vi "Custom Error Codes.vi"(8 "error in":errorcluster, 10 "PAR1":string, 11 "Enum":T1) -> (0 "error out":errorcluster)   [LabVIEW 2013, in "GOLPI library.lvlib"]
uses:
  GOLPI library.lvlib
  Custom Error Codes Enum Type Def.vi
  <vilib>/Utility/error.llb/Error Cluster From Error Code.vi
  <vilib>/ErrorRing/Error Ring.xnode
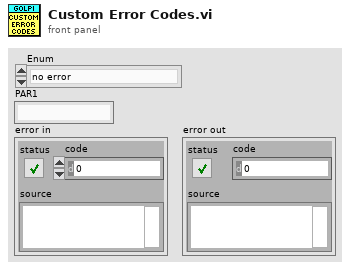
[diagram p1: front panel]
types:
  T1 = typedef "GOLPI library.lvlib/Custom Error Codes Enum Type Def.vi" = enum16{"no error", "00 working directory PAR1 missing", "01 octave binary PAR1 missing", "02 octave report error PAR1", "03 empty output last cmd PAR1", "10 var PAR1 not string", "11 var PAR1 not num, scal, ~compl", "12 var PAR1 not num, scal, compl", "13 var PAR1 not num, vect, ~compl", "14 var PAR1 not num, vect, compl"}
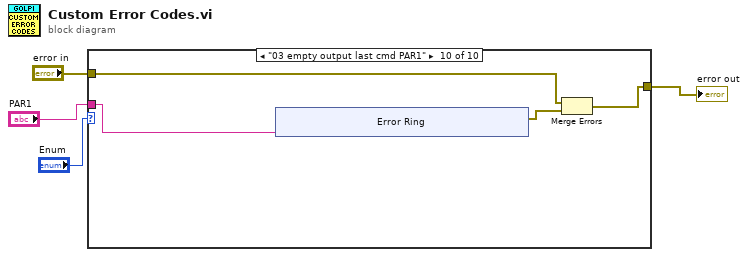
[diagram p0: block diagram]
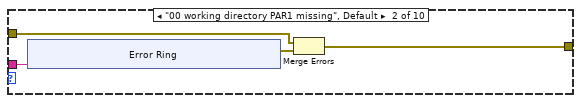
[diagram p3: hidden frame]
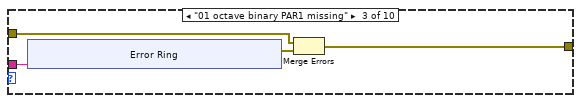
[diagram p4: hidden frame]
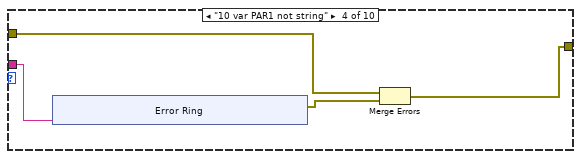
[diagram p5: hidden frame]
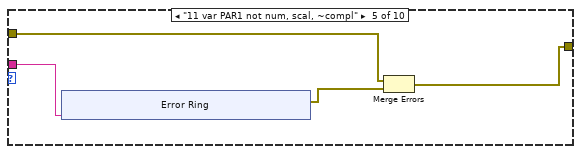
[diagram p6: hidden frame]
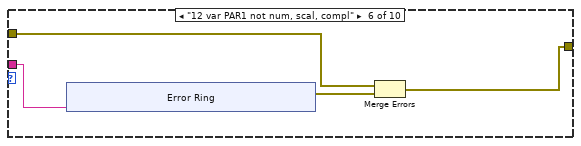
[diagram p7: hidden frame]
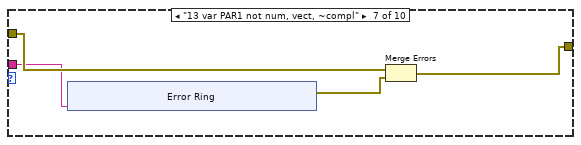
[diagram p8: hidden frame]
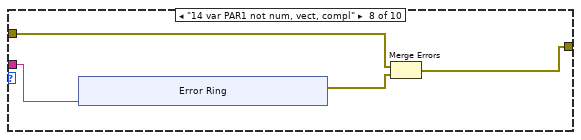
[diagram p9: hidden frame]
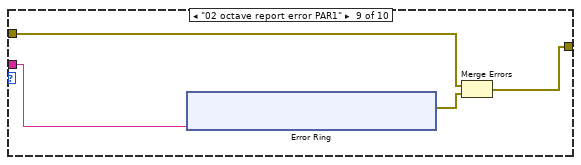
[diagram p10: hidden frame]
diagram:
  n1 = case shown="\"03 empty output last cmd PAR1\"" "Enum" {
    tunnel: "PAR1" -> [_ w9 w20 w28 w39 w51 w61 w73 w84 w97]
    tunnel: [w5 w7 w18 w29 w40 w50 w63 w72 w83 w94] -> w1
    tunnel: "error in" -> [w5 w6 w17 w30 w41 w53 w64 w74 w85 w95]
    frame "no error" {
    }
    frame "00 working directory PAR1 missing", Default {
      n2 = xnode "Error Ring"("parameter 0"=w9) -> ("error out"=w8:errorcluster)
      n3 = Merge Errors(w6, w8) -> (w7:errorcluster)
    }
    frame "01 octave binary PAR1 missing" {
      n4 = xnode "Error Ring"("parameter 0"=w20) -> ("error out"=w19:errorcluster)
      n5 = Merge Errors(w17, w19) -> (w18:errorcluster)
    }
    frame "10 var PAR1 not string" {
      n6 = xnode "Error Ring"("parameter 0"=w28) -> ("error out"=w31:errorcluster)
      n7 = Merge Errors(w30, w31) -> (w29:errorcluster)
    }
    frame "11 var PAR1 not num, scal, ~compl" {
      n8 = xnode "Error Ring"("parameter 0"=w39) -> ("error out"=w42:errorcluster)
      n9 = Merge Errors(w41, w42) -> (w40:errorcluster)
    }
    frame "12 var PAR1 not num, scal, compl" {
      n10 = xnode "Error Ring"("parameter 0"=w51) -> ("error out"=w52:errorcluster)
      n11 = Merge Errors(w53, w52) -> (w50:errorcluster)
    }
    frame "13 var PAR1 not num, vect, ~compl" {
      n12 = xnode "Error Ring"("parameter 0"=w61) -> ("error out"=w62:errorcluster)
      n13 = Merge Errors(w64, w62) -> (w63:errorcluster)
    }
    frame "14 var PAR1 not num, vect, compl" {
      n14 = xnode "Error Ring"("parameter 0"=w73) -> ("error out"=w75:errorcluster)
      n15 = Merge Errors(w74, w75) -> (w72:errorcluster)
    }
    frame "02 octave report error PAR1" {
      n16 = xnode "Error Ring"("parameter 0"=w84) -> ("error out"=w86:errorcluster)
      n17 = Merge Errors(w85, w86) -> (w83:errorcluster)
    }
    frame "03 empty output last cmd PAR1" {
      n18 = xnode "Error Ring"("parameter 0"=w97) -> ("error out"=w96:errorcluster)
      n19 = Merge Errors(w95, w96) -> (w94:errorcluster)
    }
  }
  "error out" <- w1
